vi "Configure Measurement (Frequency Ratio).vi"(5 "Ratio Estimate (1)":dbl=1.0 format="%^#_6g", 7 "Ratio Resolution (0.001)":dbl=0.001, 8 "error in (no error)":errorcluster, 9 "Denominator Frequency Channel (2:Channel 2)":i32(ring)=2 items=["Channel 1"=1, "Channel 2"=2, "Channel 3"=3], 10 "Numerator Frequency Channel (1:Channel 1)":i32(ring)=1 items=["Channel 1"=1, "Channel 2"=2, "Channel 3"=3], 11 "VISA resource name":refnum<visa-resource-name>) -> (0 "error out":errorcluster, 3 "VISA resource name out":refnum<visa-resource-name>)   [LabVIEW 2024, in "Agilent 532XX Series.lvlib"]
doc: "Configures settings required for Frequency Ratio Measurements."
uses:
  Agilent 532XX Series.lvlib
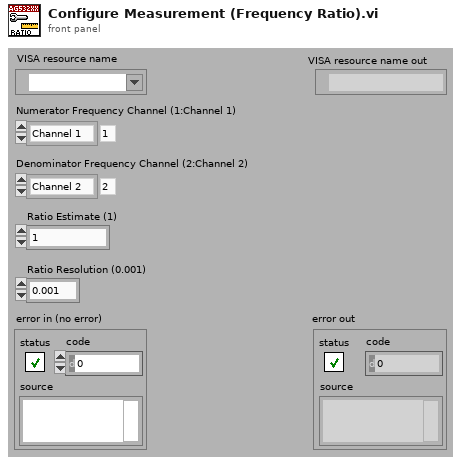
[diagram p1: front panel]
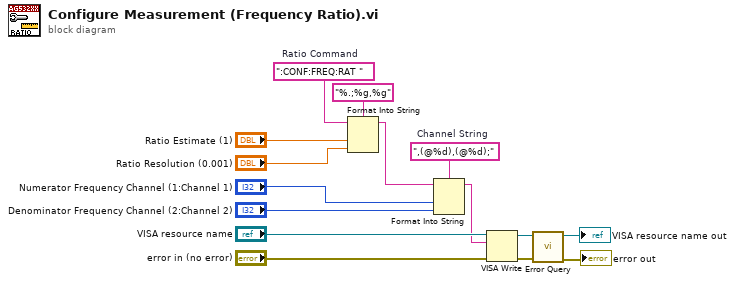
[diagram p0: block diagram]
diagram:
  w4 = ",(@%d),(@%d);"  # Channel String
  w8 = ":CONF:FREQ:RAT "  # Ratio Command
  n1 = Format Into String(format string="%.;%g,%g" ("Ratio Command"), initial string=w8, "Ratio Estimate (1)", "Ratio Resolution (0.001)") -> (resulting string=w5:string)  [unwired: 1 in, 1 out]
  n2 = Format Into String(format string=w4, initial string=w5, "Numerator Frequency Channel (1:Channel 1)", "Denominator Frequency Channel (2:Channel 2)") -> (resulting string=w3:string)  [unwired: 1 in, 1 out]
  n3 = VISA Write(VISA resource name="VISA resource name", write buffer=w3, error in (no error)="error in (no error)") -> (VISA resource name out=w10:refnum<visa-resource-name>, error out=w12:errorcluster)  [unwired: 1 out]
  n4 = call "Error Query.vi"("error in (no error)"=w12, "VISA resource name"=w10) -> ("error out"=→"error out":errorcluster, "VISA resource name out"=→"VISA resource name out":refnum<visa-resource-name>)  [unwired: 8 out]
